vi "Advance past next JSON Value (inlined COPY).vi"(7 "JSON":string, 9 "Offset":i32, 11 "State":T1=enum."Leading Whitespace") -> (1 "Offset":i32, 3 "State":T1=enum."Value end", 4 "Type":T1, 6 "Value start":i32)   [LabVIEW 2015, in "JSONtext.lvlib"]
uses:
  JSONtext.lvlib
  Parsing State.ctl
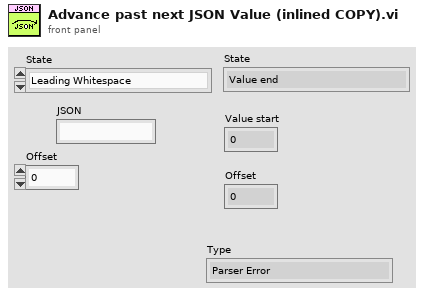
[diagram p1: front panel]
types:
  T1 = typedef "JSONtext.lvlib/Parsing State.ctl" = enum16{"Parser Error", "Object", "Array", "String", "Number/Other", "Leading Whitespace", "Object end", "Array end", "Value end"}
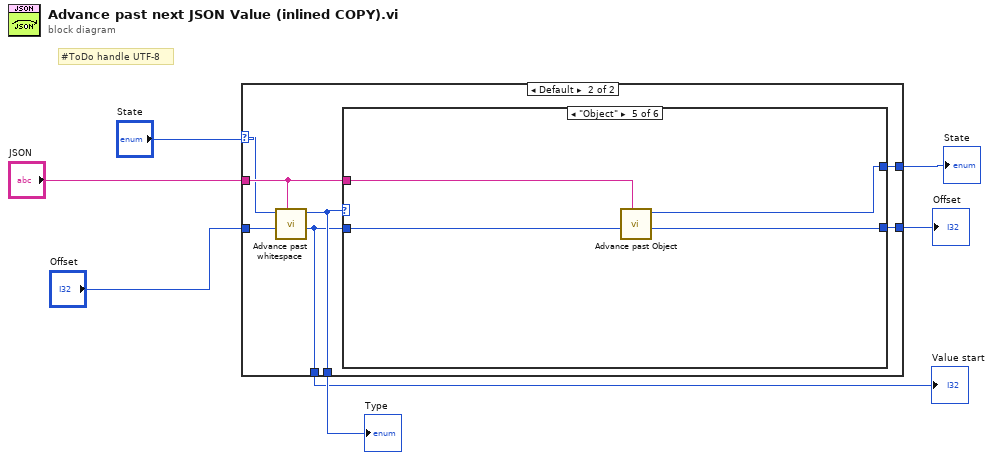
[diagram p0: block diagram]
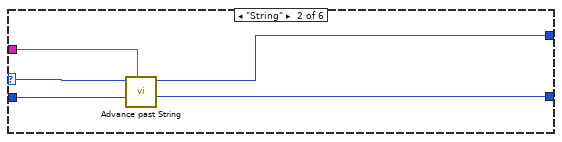
[diagram p4: hidden frame]
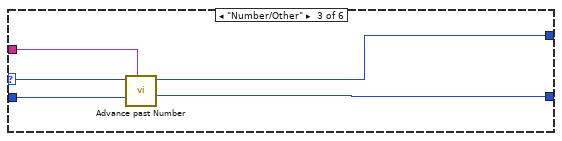
[diagram p5: hidden frame]
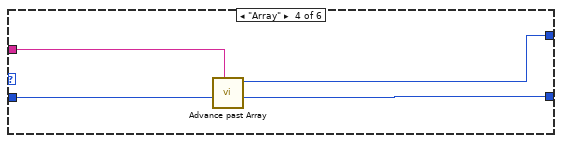
[diagram p6: hidden frame]
diagram:
  # "#ToDo handle UTF-8"
  n1 = case shown="Default" "State" {
    selector: "State" -> [w8 w10]
    tunnel: "JSON" -> [_ w16]
    tunnel: [w8 w15] -> w6
    tunnel: [w9 w14] -> w5
    tunnel: [w8 w13] -> w4
    tunnel: "Offset" -> [w9 w12]
    tunnel: [w9 w11] -> w2
    frame "Parser Error" {
    }
    frame Default {
      n2 = call "Advance past whitespace.vi"("JSON"=w16, "Offset"=w12, "Parser State in"=w10) -> ("Offset of first non-whitespace"=w11:i32, "Parser State"=w15:T1)  [unwired: 7 in]
      n3 = case shown="\"Object\"" w15 {
        selector: w15 -> [w17 w22 w27 _ _ w37]
        tunnel: w16 -> [_ w23 w28 w29 w33 _]
        tunnel: w11 -> [w18 w21 w26 w30 w36 w38]
        tunnel: [w18 w20 w25 w31 w34 w38] -> w14
        tunnel: [w17 w19 w24 w32 w35 w37] -> w13
        frame "Parser Error", Default {
        }
        frame "String" {
          n4 = call "Advance past String.vi"("JSON"=w23, "Offset"=w21, "State in"=w22) -> ("Offset past match"=w20:i32, "State"=w19:T1)  [unwired: 6 in, 1 out]
        }
        frame "Number/Other" {
          n5 = call "Advance past Number.vi"("JSON"=w28, "Offset (0)"=w26, "Parser State in"=w27) -> ("Offset past match"=w25:i32, "Parser State"=w24:T1)  [unwired: 6 in, 1 out]
        }
        frame "Array" {
          n6 = call "Advance past Array.vi"("JSON"=w29, "Offset"=w30) -> ("Offset past Array"=w31:i32, "State"=w32:T1)  [unwired: 7 in, 1 out]
        }
        frame "Object" {
          n7 = call "Advance past Object.vi"("JSON"=w33, "Offset"=w36) -> ("Offset past Object"=w34:i32, "State"=w35:T1)  [unwired: 7 in, 1 out]
        }
        frame "Value end" {
          # "null, true, etc."
        }
      }
    }
  }
  "State" <- w4
  "Offset" <- w5
  "Value start" <- w2
  "Type" <- w6
